vi "Test Senders are Not Presented as Processes.vi"(8 "error in (no error)":errorcluster, 11 "Test Case In":refnum<class "Processes List View Model Test.lvclass">) -> (0 "error out":errorcluster, 3 "Test Case Out":refnum<class "Processes List View Model Test.lvclass">)   [LabVIEW 2020, in "Processes List View Model Test.lvclass"]
uses:
  Processes List View Model Test.lvclass
  Processes List View Model Test.lvclass/Processes List View Model Test.ctl
  01074fa8-ee8a-411d-bc8b-fc92c4f90959.vi
  source/List Box View Model_/List Box View Model.lvclass
  source/Debug Data/Debug Data.lvclass
  source/Debug Data/Raw Debug Data.ctl
  source/List Seen Processes View Model/List Processes View Model.lvclass
  C:/Git/astemes-triarc-debugger/source/List Box View Model_/List Box View Model.lvclass
  C:/Git/astemes-triarc-debugger/source/List Seen Processes View Model/List Processes View Model.lvclass
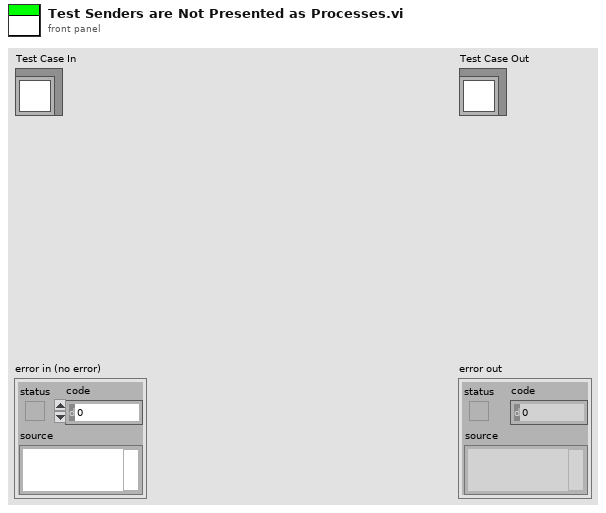
[diagram p1: front panel]
types:
  T1 = typedef "Debug Data.lvclass/Raw Debug Data.ctl" = cluster{"Action":string, "Call Chain":string, "Process":string, "Message":string, "Message Data":variant, "Time":dbl}
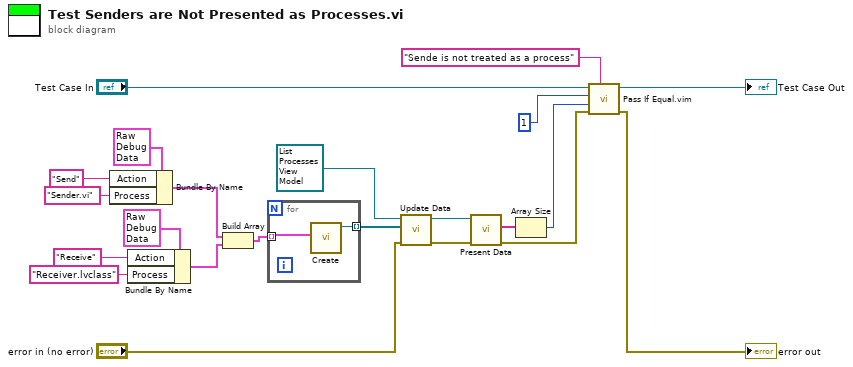
[diagram p0: block diagram]
diagram:
  n1 = Bundle By Name(cluster=T1 {"Action"="", "Call Chain"="", "Process"="", "Message"="", "Message Data"=variant, "Time"=0.0} ("Debug Data Cluster"), "Action"="Send", "Process"="Sender.vi") -> (w17:T1)
  n2 = Bundle By Name(cluster=T1 {"Action"="", "Call Chain"="", "Process"="", "Message"="", "Message Data"=variant, "Time"=0.0} ("Debug Data Cluster"), "Action"="Receive", "Process"="Receiver.lvclass") -> (w10:T1)
  n3 = Build Array(w17, w10) -> (w14:T1[])
  n4 = for {
    tunnel: w14 -> [w24] mode=indexing
    tunnel: [w23] -> w18 mode=indexing
    n5 = call "Create.vi"("Debug Data Cluster"=w24) -> ("Debug Data out"=w23:refnum<class "Debug Data.lvclass">)  [unwired: 9 in, 1 out]
  }
  n6 = call-dynamic "Update Data.vi"("error in (no error)"="error in (no error)", "Debug Data"=w18, "List Seen Processes View Model In"=refnum<class "List Processes View Model.lvclass"> refnum) -> ("error out"=w20:errorcluster, "List Seen Processes View Model Out"=w21:refnum<class "List Processes View Model.lvclass">)  [unwired: 7 in]
  n7 = call "Present Data.vi"("error in (no error)"=w20, "List Seen Processes View Model In"=w21) -> ("error out"=w5:errorcluster, "Message List"=w9:string[])  [unwired: 7 in, 1 out]
  n8 = Array Size(array=w9) -> (size(s)=w6:i32)
  n9 = call "Pass If Equal.vim"("Description"="Sende is not treated as a process", "error in (no error)"=w5, "Actual"=w6, "Expected"=1 ("size(s)"), "LUnit Test Case In"="Test Case In") -> ("error out"=→"error out":errorcluster, "LUnit Test Case Out"=→"Test Case Out":refnum<class "Processes List View Model Test.lvclass">)  [unwired: 5 in]
